vi "number display.vi"() -> ()   [LabVIEW 2020]
panel:
  out "transposed array":bool[][](array[boolean])
  in  "Numeric":dbl min=0.0 max=9999.0 format="%#_13g"
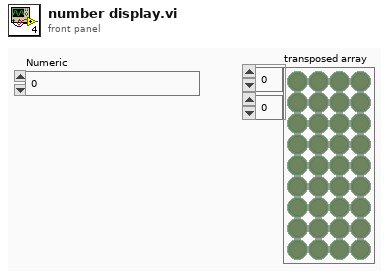
[diagram p1: front panel]
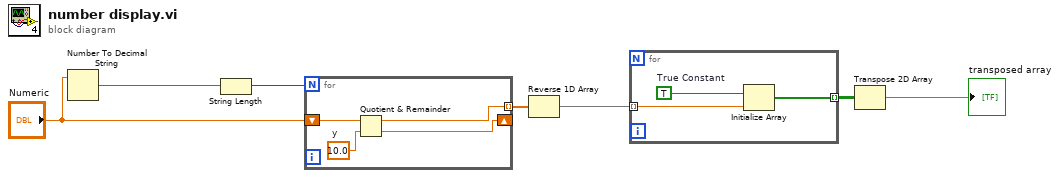
[diagram p0: block diagram]
diagram:
  n1 = Number To Decimal String(number="Numeric") -> (decimal integer string=w6:string)  [unwired: 1 in]
  n2 = String Length(string=w6) -> (length=w7:i32)
  n3 = for {
    N: w7 -> [_]
    shift-right: [w9] -> _
    shift-left: "Numeric" -> [w11]
    tunnel: [w8] -> w4 mode=indexing
    w10 = 10.0  # y
    n4 = Quotient & Remainder(x=w11, y=w10) -> (x-y*floor(x/y)=w8:dbl, floor(x/y)=w9:dbl)
  }
  n5 = Reverse 1D Array(array=w4) -> (reversed array=w3:dbl[])
  n6 = for {
    tunnel: w3 -> [w14] mode=indexing
    tunnel: [w12] -> w2 mode=indexing
    w13 = TRUE  # True Constant
    n7 = Initialize Array "Initialize Array"(w13, w14) -> (w12:bool[])
  }
  n8 = Transpose 2D Array(2D array=w2) -> (transposed array=→"transposed array":bool[][])
